vi "Set UI Control Value.vi"(8 "error in (no error)":errorcluster, 10 "VI Ref":refnum<vi>, 11 "Boolean Parameter in":refnum<class "File Path Parameter.lvclass">) -> (0 "error out":errorcluster, 3 "Boolean Parameter out":refnum<class "File Path Parameter.lvclass">)   [LabVIEW 2019, in "CD Parameter Manager API.lvlib" / "File Path Parameter.lvclass"]
uses:
  File Path Parameter.lvclass
  C:/Repositories/UI-Control-Initializer-API/Source/Parameter Class/Parameter.lvclass
  Parameter Class/Parameter.lvclass/Parameter.ctl
  File Path Parameter.lvclass/File Path Parameter.ctl
  Parameter Class/Member Accessors/Read Control label.vi
  Member Accessors/Read Value.vi
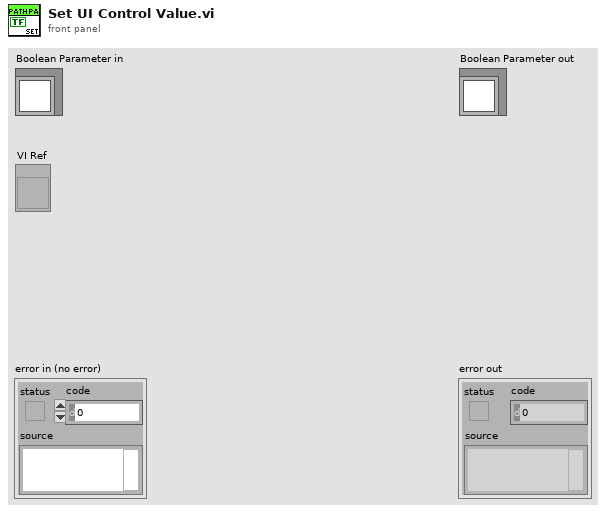
[diagram p1: front panel]
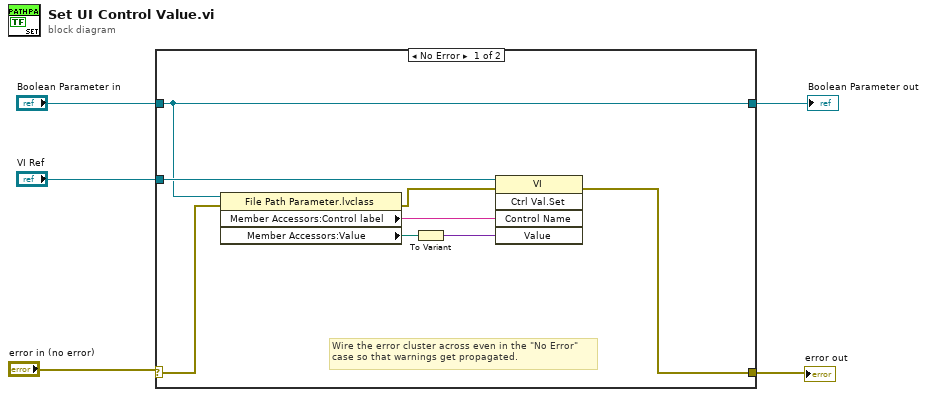
[diagram p0: block diagram]
diagram:
  n1 = case shown="No Error" "error in (no error)" {
    selector: "error in (no error)" -> [w7 w15]
    tunnel: [w13 w15] -> w3
    tunnel: "VI Ref" -> [w12 _]
    tunnel: [w11 w14] -> w4
    tunnel: "Boolean Parameter in" -> [w11 w14]
    frame No Error {
      # "Wire the error cluster across even in the \"No Error\"\ncase so that warnings get propagated."
      n2 = property class="File Path Parameter.lvclass"(reference=w11, error in=w7) -> (error out=w6:errorcluster, "Member Accessors:Control label"=w8:string, "Member Accessors:Value"=w9:path)  [unwired: 1 out]
      n3 = To Variant(anything=w9) -> (Variant=w10:variant)
      n4 = invoke class="VI" method="Ctrl Val.Set"(reference=w12, error in=w6, "Control Name"=w8, "Value"=w10) -> (error out=w13:errorcluster)  [unwired: 1 in, 4 out]
    }
    frame Error {
    }
  }
  "error out" <- w3
  "Boolean Parameter out" <- w4
